vi "Create table if not exists.vi"(8 "error in (no error)":errorcluster, 11 "IConfigDBQueries in":refnum<class "mysql-queries.lvclass">) -> (0 "error out":errorcluster, 2 "Query out":string)   [LabVIEW 2020, in "mysql-queries.lvlib" / "mysql-queries.lvclass"]
uses:
  mysql-queries.lvclass
  mysql-queries.lvclass/mysql-queries.ctl
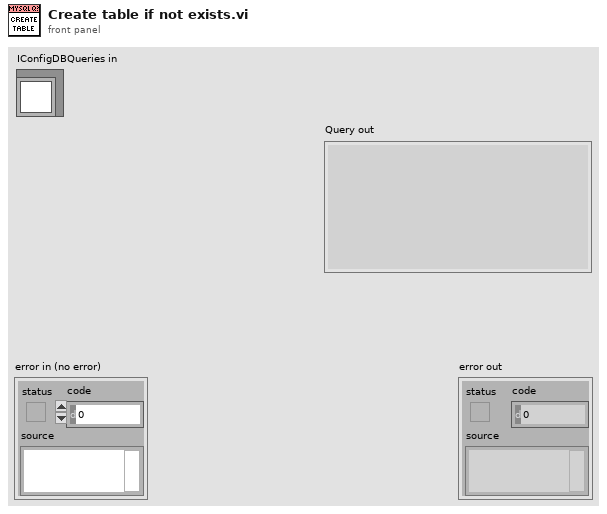
[diagram p1: front panel]
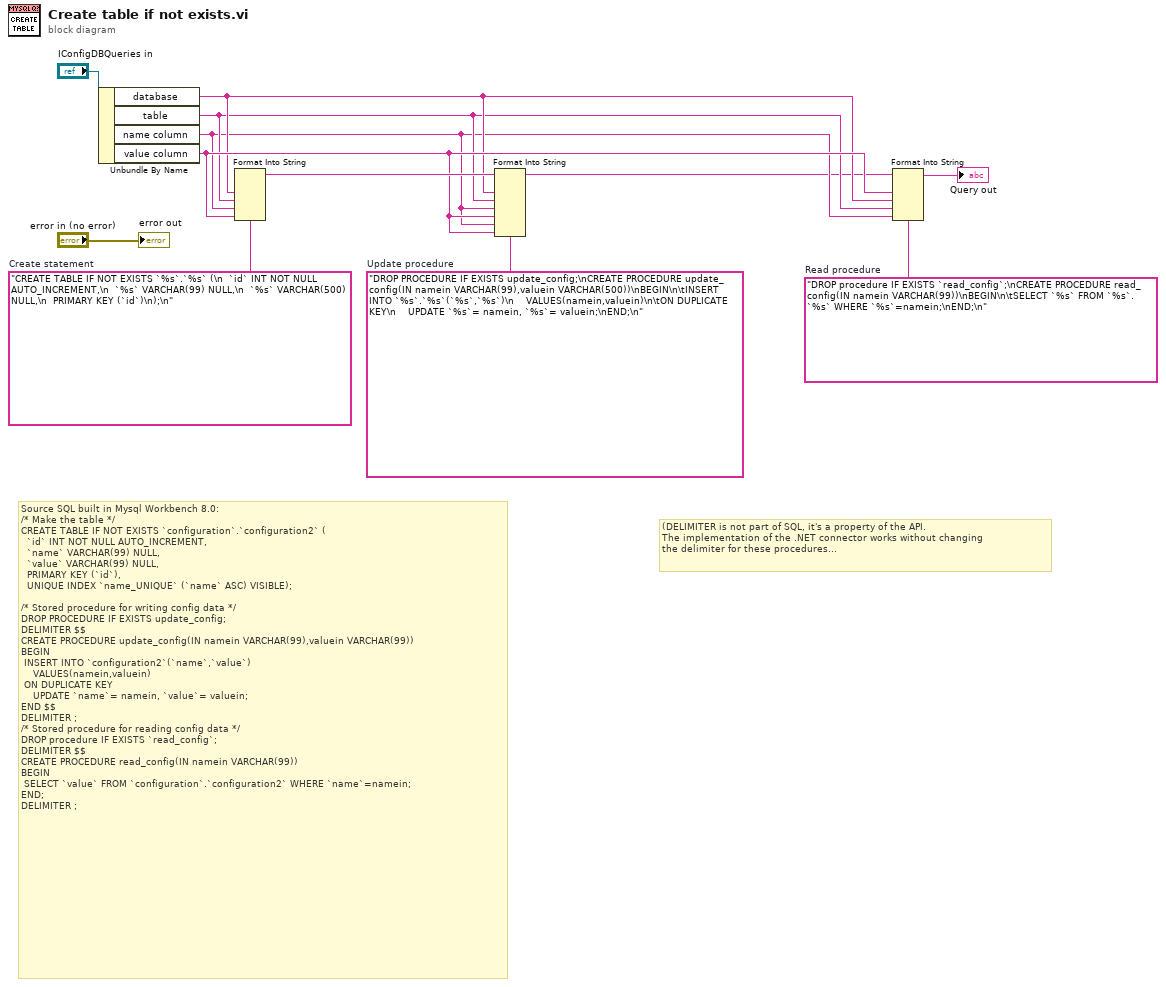
[diagram p0: block diagram]
diagram:
  w8 = "DROP procedure IF EXISTS `read_config`;\nCREATE PROCEDURE read_config(IN namein VARCHAR(99))\nBEGIN\n\tSELECT `%s` FROM `%s`.`%s` WHERE `%s`=namein;\nEND;\n"  # Read procedure
  w9 = "DROP PROCEDURE IF EXISTS update_config;\nCREATE PROCEDURE update_config(IN namein VARCHAR(99),valuein VARCHAR(500))\nBEGIN\n\tINSERT INTO `%s`.`%s`(`%s`,`%s`)\n    VALUES(namein,valuein)\n\tON DUPLICATE KEY\n    UPDATE `%s`= namein, `%s`= valuein;\nEND;\n"  # Update procedure
  w11 = "CREATE TABLE IF NOT EXISTS `%s`.`%s` (\n  `id` INT NOT NULL AUTO_INCREMENT,\n  `%s` VARCHAR(99) NULL,\n  `%s` VARCHAR(500) NULL,\n  PRIMARY KEY (`id`)\n);\n"  # Create statement
  # "(DELIMITER is not part of SQL, it's a property of the API.\nThe implementation of the .NET connector works without changing\nthe delimiter for these procedures..."
  # "Source SQL built in Mysql Workbench 8.0:\n/* Make the table */\nCREATE TABLE IF NOT EXISTS `configuration`.`configuration2` (\n  `id` INT NOT NULL AUTO_INCREMENT,\n  `name` VARCHAR(99) NULL,\n  `value` VARCHAR(99) NULL,\n  PRIMARY KEY (`id`),\n  UNIQUE INDEX `name_UNIQUE` (`name` ASC) VISIBLE);\n\n/* Stored procedure for writing config data */\nDROP PROCEDURE IF EXISTS update_config;\nDELIMITER $$\nCREATE PROCEDURE update_config(IN namein VARCHAR(99),valuein VARCHAR(99))\nBEGIN\n\tINSERT INTO `configuration2`(`name`,`value`)\n    VALUES(namein,valuein)\n\tON DUPLICATE KEY\n    UPDATE `name`= namein, `value`= valuein;\nEND $$\nDELIMITER ;\n/* Stored procedure for reading config data */\nDROP procedure IF EXISTS `read_config`;\nDELIMITER $$\nCREATE PROCEDURE read_config(IN namein VARCHAR(99))\nBEGIN\n\tSELECT `value` FROM `configuration`.`configuration2` WHERE `name`=namein;\nEND;\nDELIMITER ;"
  n1 = Unbundle By Name("IConfigDBQueries in") -> ("database"=w6:string, "table"=w5:string, "name column"=w4:string, "value column"=w7:string)
  n2 = Format Into String(format string=w11, w6, w5, w4, w7) -> (resulting string=w10:string)  [unwired: 2 in, 1 out]
  n3 = Format Into String(format string=w9, initial string=w10, w6, w5, w4, w7, w4, w7) -> (resulting string=w3:string)  [unwired: 1 in, 1 out]
  n4 = Format Into String(format string=w8, initial string=w3, w7, w6, w5, w4) -> (resulting string=→"Query out":string)  [unwired: 1 in, 1 out]
  "error out" <- "error in (no error)"
